vi "Search Packages by String.vi"(7 "Package Search Options":T1={"Include GPM"=TRUE, "Include VIPM"=TRUE, "Include NIPM"=TRUE}, 8 "error in (no error)":errorcluster, 10 "Search String":string, 11 "GCentral API in":refnum<class "GCentral API.lvclass">) -> (0 "error out":errorcluster, 2 "Packages":refnum<class "Package.lvclass">[](array[class]), 3 "GCentral API out":refnum<class "GCentral API.lvclass">, 4 "Debug Link":string)   [LabVIEW 2020, in "GCentral-API.lvlib" / "GCentral API.lvclass"]
uses:
  GCentral API.lvclass
  Package Search Options.ctl
  Package/Package.lvclass
  search-json.ctl
  API Endpoint.ctl
  GCentral-API.lvlib
  neg-pkg/JSON/JSON.lvlib
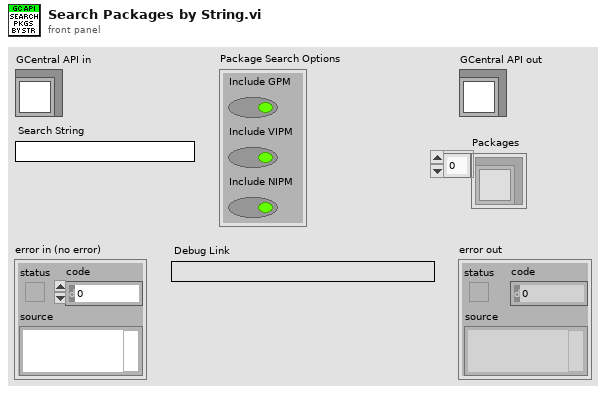
[diagram p1: front panel]
types:
  T1 = typedef "GCentral-API.lvlib/Package Search Options.ctl" = cluster{"Include GPM":bool, "Include VIPM":bool, "Include NIPM":bool}
  T2 = typedef "GCentral-API.lvlib/API Endpoint.ctl" = enum16{"packages/list", "packages/search"}
  T3 = typedef "GCentral-API.lvlib/search-json.ctl" = cluster{"terms":string[], "repos":cluster{"gpm":bool, "vipm":bool, "nipm":bool}}
  T4 = typedef "JSON.lvlib/JSON Item Type.ctl" = enum16{"unknown", "null", "Array", "Object", "String", "Number", "Boolean"}
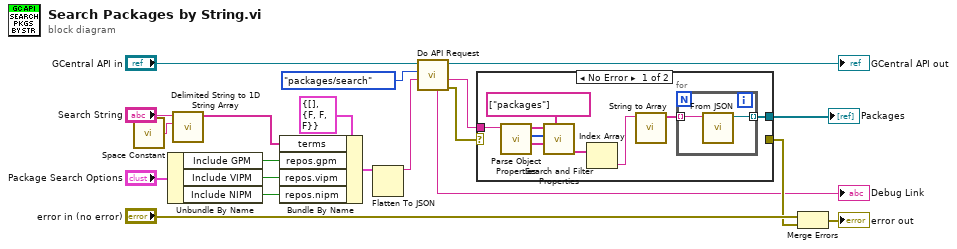
[diagram p0: block diagram]
diagram:
  n1 = call <vilib>:"Space Constant.vi"() -> ("String"=w17:string)
  n2 = Unbundle By Name("Package Search Options") -> ("Include GPM"=w14:bool, "Include VIPM"=w13:bool, "Include NIPM"=w12:bool)
  n3 = call <vilib>:"Delimited String to 1D String Array.vi"("delimiter"=w17, "delimited string"="Search String") -> ("string array"=w15:string[])  [unwired: 9 in]
  n4 = Bundle By Name(cluster=T3 {"terms"=[], "repos"={"gpm"=FALSE, "vipm"=FALSE, "nipm"=FALSE}} ("search-json"), "terms"=w15, "repos.gpm"=w14, "repos.vipm"=w13, "repos.nipm"=w12) -> (w11:T3)
  n5 = Flatten To JSON(anything=w11) -> (JSON string=w4:string)  [unwired: 2 in, 1 out]
  n6 = call "Do API Request.vi"("Payload (Empty = GET, payload = POST)"=w4, "API Endpoint"=API_Endpoint."packages/search", "GCentral API in"="GCentral API in") -> ("error out"=w3:errorcluster, "Response"=w2:string, "GCentral API out"=→"GCentral API out":refnum<class "GCentral API.lvclass">, "Debug Link"=→"Debug Link":string)  [unwired: 4 in, 1 out]
  n7 = case shown="No Error" w3 {
    selector: w3 -> [_ w32]
    tunnel: w2 -> [w23 _]
    tunnel: [w21 _] -> w8
    tunnel: [_ w32] -> w9
    frame No Error {
      n8 = call "Parse Object Properties.vi"("JSON String"=w23) -> ("Values"=w27:string[], "Item Types"=w28:T4[], "Keys"=w29:string[])  [unwired: 7 in, 1 out]
      n9 = call "Search and Filter Properties.vi"("Search Keys"=string[] ["packages"], "Values In"=w27, "Types In"=w28, "Keys In"=w29) -> ("Filtered Values"=w25:string[])  [unwired: 2 in, 5 out]
      n10 = Index Array(array=w25) -> (element=w24:string)  [unwired: 1 in]
      n11 = call "String to Array.vi"("Array String In"=w24) -> ("JSON Strings"=w22:string[])  [unwired: 10 in]
      n12 = for {
        tunnel: w22 -> [w31] mode=indexing
        tunnel: [w30] -> w21 mode=indexing
        n13 = call "From JSON.vi"("JSON"=w31) -> ("Package out"=w30:refnum<class "Package.lvclass">)  [unwired: 9 in, 1 out]
      }
    }
    frame Error {
    }
  }
  "Packages" <- w8
  n14 = Merge Errors("error in (no error)", w9) -> (→"error out":errorcluster)
